vi "Check Status of Saving to Save Area.vi"(8 "error in (no error)":errorcluster {"code" format="%.0x"}, 11 "Device ID (0)":i32) -> (0 "error out":errorcluster {"code" format="%.0x"}, 2 "Busy":bool, 3 "Device ID out":i32)   [LabVIEW 2020, in "KEYENCE LJ-X8000A.lvlib"]
doc: "This function checks whether the controller is accessing the save area with an operation\nsuch as that to save settings.\nWhen the controller was instructed to save settings to the save area with the\n<B>Return to Factory Setting</B> VI, <B>Set Setting</B> VI, <B>Initialize Setting</B> VI, \nor the <B>Reflect Setting</B> VI, \ncheck that access to the save area has completed with this function before turning off the power."
uses:
  KEYENCE LJ-X8000A.lvlib
panel:
  # "(c) 2019 KEYENCE CORPORATION.  ALL RIGHTS RESERVED."
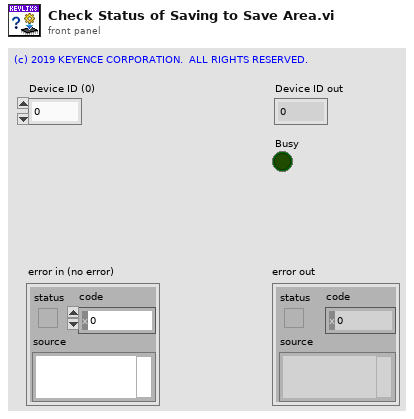
[diagram p1: front panel]
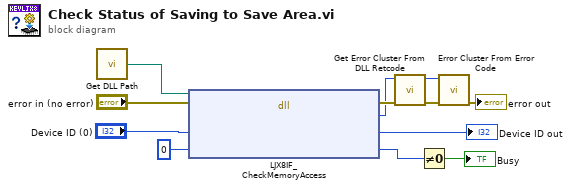
[diagram p0: block diagram]
diagram:
  n1 = call "Get DLL Path.vi"() -> ("DLL Path"=w9:path)  [unwired: 3 in]
  n2 = dll-call lib="C:/Program Files (x86)/National Instruments/LabVIEW 2018/instr.lib/KEYENCE LJ-X8000/LJX8_IF.*" fn="LJX8IF_CheckMemoryAccess"(path in=w9, error in="error in (no error)", "lDeviceId"="Device ID (0)", "pbyBusy"=u8 0) -> (error out=w7:errorcluster, "lRetCode"=w6:i32, "lDeviceId"=→"Device ID out":i32, "pbyBusy"=w4:u8)  [unwired: 1 in, 1 out]
  n3 = call "Get Error Cluster From DLL Retcode.vi"("error in (no error)"=w7, "DLL Return Code"=w6) -> ("error out"=w8:errorcluster, "VI Error Code"=w1:i32)  [unwired: 8 in]
  n4 = Not Equal To 0?(x=w4) -> (x != 0?=→"Busy":bool)
  n5 = call <vilib>:"Error Cluster From Error Code.vi"("error in (no error)"=w8, "error code (0)"=w1) -> ("error out"=→"error out":errorcluster)  [unwired: 7 in]
